vi "Report_generator.vi"() -> ()   [LabVIEW 2022 SP3]
uses:
  <vilib>/printing/EasyPrintingControls.llb/custom_contents_options.ctl
  <vilib>/printing/EasyPrintingControls.llb/list_which_controls.ctl
  <vilib>/Utility/NIReport.llb/Report Type.ctl
  <vilib>/printing/EasyPrintingControls.llb/contents.ctl
  <vilib>/Utility/NIReport.llb/Report Type (with Quick Print).ctl
  <vilib>/printing/EasyPrinting.llb/Print VI Panel or Documentation (path).vi
  <vilib>/Utility/NIReport.llb/Append Report Text (str wrap).vi
  <vilib>/printing/ReportDocExtensions.llb/Append VI Icon to Report (refnum).vi
  <vilib>/printing/ReportDocExtensions.llb/Append VI Description to Report (refnum).vi
  <vilib>/printing/ReportDocExtensions.llb/Append Front Panel Image to Report (refnum).vi
  <vilib>/printing/ReportDocExtensions.llb/Append VI List of Controls to Report (refnum).vi
  <vilib>/printing/ReportDocExtensions.llb/Append VI List of SubVIs to Report (refnum).vi
  <vilib>/printing/ReportDocExtensions.llb/Append VI Hierarchy to Report (refnum).vi
  <vilib>/Utility/NIReport.llb/NI_report.lvclass
  <vilib>/Utility/NIReport.llb/NI_ReportGenerationCore.lvlib
panel:
  out "error out 2":errorcluster
  in  "custom contents options":T1 {"list of controls options"."list which controls?" items=["all controls", "connected controls"]}
  in  "VI path":path
  out "error out":errorcluster
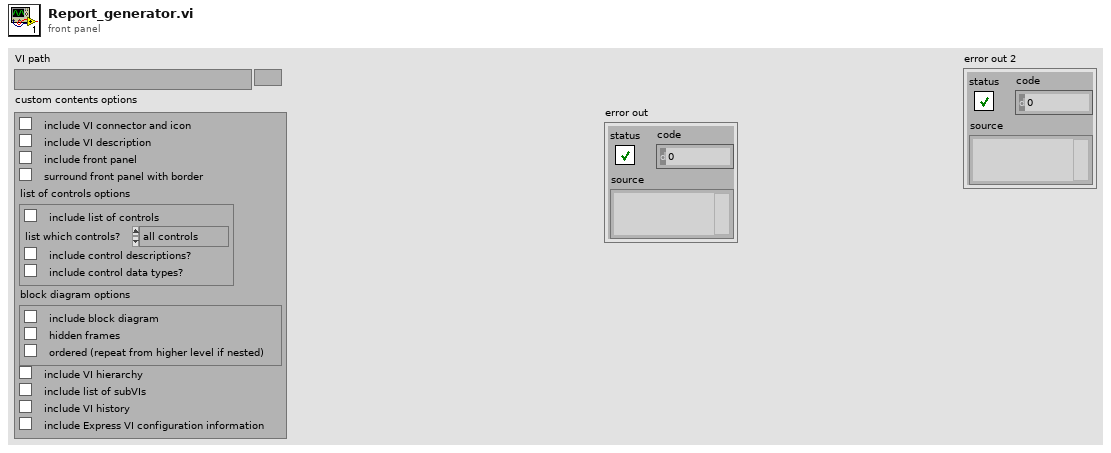
[diagram p1: front panel]
types:
  T1 = typedef "NI_ReportGenerationCore.lvlib/custom_contents_options.ctl" = cluster{"include VI connector and icon":bool, "include VI description":bool, "include front panel":bool, "surround front panel with border":bool, "list of controls options":cluster{"include list of controls":bool, "list which controls?":T2, "include control descriptions?":bool, "include control data types?":bool}, "block diagram options":cluster{"include block diagram":bool, "hidden frames":bool, "ordered (repeat from higher level if nested)":bool}, "include VI hierarchy":bool, "include list of subVIs":bool, "include VI history":bool, "include Express VI configuration information":bool}
  T2 = typedef "NI_ReportGenerationCore.lvlib/list_which_controls.ctl" = u16
  T3 = typedef "NI_ReportGenerationCore.lvlib/Report Type (with Quick Print).ctl" = enum16{"Quick Print", "HTML", "Word", "Excel"}
  T4 = typedef "NI_ReportGenerationCore.lvlib/contents.ctl" = u16
  T5 = typedef "NI_ReportGenerationCore.lvlib/Report Type.ctl" = enum16{"HTML", "Word", "Excel"}
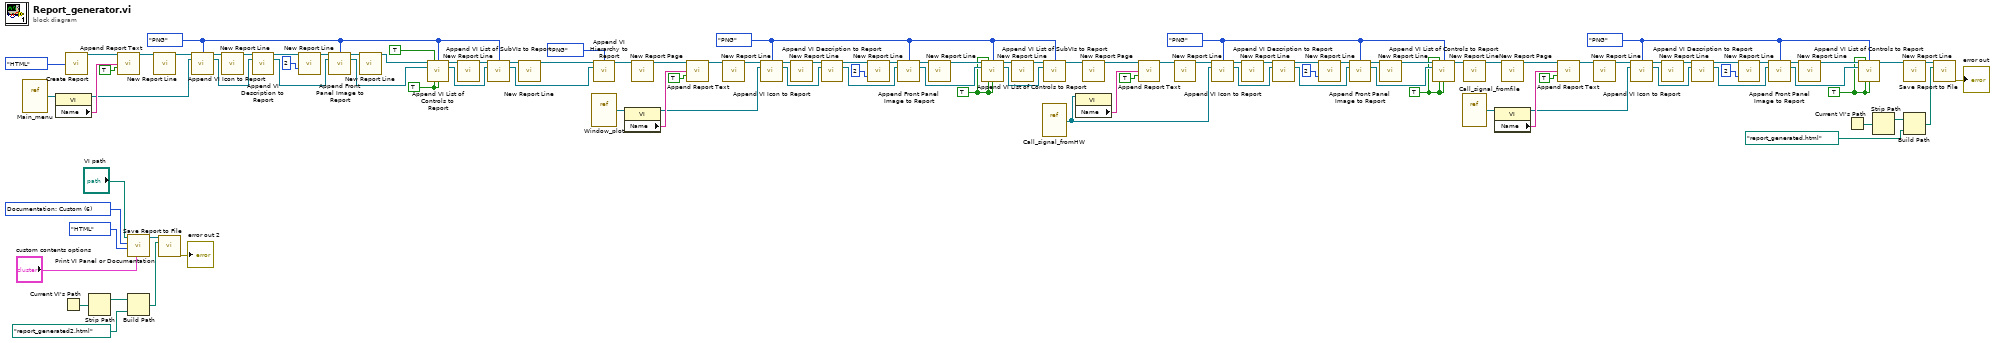
[diagram p0: block diagram]
diagram:
  w9 = T4 6 items=["Complete front panel", "Visible portion of front panel", "Icon, description, panel and diagram", "Documentation: Using the panel", "Documentation: Using as a subVI", "Documentation: Complete", "Documentation: Custom"] ("contents (complete front panel)")
  w12 = enum32{"PNG", "JPEG", "GIF"}."PNG" ("image format (jpeg)")
  w20 = TRUE ("include only controls in con pane?")
  w13 = enum32{"PNG", "JPEG", "GIF"}."PNG" ("image format (jpeg)")
  w21 = TRUE ("include only controls in con pane?")
  w14 = enum32{"PNG", "JPEG", "GIF"}."PNG" ("image format (jpeg)")
  w22 = TRUE ("include only controls in con pane?")
  w15 = enum32{"PNG", "JPEG", "GIF"}."PNG" ("image format (jpeg)")
  w23 = TRUE ("include only controls in con pane?")
  n1 = vi-ref "Main_menu.vi"() -> (w82:refnum<vi>)
  n2 = property class="VI"(reference=w82) -> (reference out=w26:refnum<vi>, "Name"=w81:string)  [unwired: 1 in, 1 out]
  n3 = Current VI's Path() -> (path=w2:path)
  n4 = call <vilib>:"Create Report.vi"("report type"=Report_Type."HTML") -> ("report out"=w107:refnum<class "NI_report.lvclass">)  [unwired: 13 in, 1 out]
  n5 = Strip Path(path=w2) -> (stripped path=w3:path)  [unwired: 1 out]
  n6 = call-poly <vilib>:"Append Report Text.vi"("report in"=w107, "text"=w81, "append on new line? (F)"=TRUE) -> ("report out"=w101:refnum<class "NI_report.lvclass">)  [unwired: 9 in, 3 out]
  n7 = call-poly <vilib>:"Print VI Panel or Documentation.vi"("custom contents options"="custom contents options", "report type (Quick Print)"=Report_Type_(with_Quick_Print)."HTML", "contents (complete front panel)"=w9, "VI path"="VI path") -> ("report out"=w1:refnum<class "NI_report.lvclass">)  [unwired: 6 in, 1 out]
  n8 = Build Path(base path=w3, name or relative path=path "report_generated2.html") -> (appended path=w5:path)
  n9 = call-dynamic "New Report Line.vi"("report in"=w101) -> ("report out"=w100:refnum<class "NI_report.lvclass">)  [unwired: 13 in, 1 out]
  n10 = call-dynamic "Save Report to File.vi"("report in"=w1, "report file path"=w5) -> ("error out"=→"error out 2":errorcluster)  [unwired: 12 in, 1 out]
  n11 = call-poly <vilib>:"Append VI Icon to Report.vi"("report in"=w100, "image format (jpeg)"=w15, "VI"=w26) -> ("report out"=w93:refnum<class "NI_report.lvclass">, "VI out"=w99:refnum<vi>)  [unwired: 8 in, 3 out]
  n12 = call-dynamic "New Report Line.vi"("report in"=w93) -> ("report out"=w94:refnum<class "NI_report.lvclass">)  [unwired: 13 in, 1 out]
  n13 = call-poly <vilib>:"Append VI Description to Report.vi"("report in"=w94, "VI"=w99) -> ("report out"=w90:refnum<class "NI_report.lvclass">, "VI out"=w98:refnum<vi>)  [unwired: 9 in, 3 out]
  n14 = call-dynamic "New Report Line.vi"("report in"=w90, "number of lines (1)"=2) -> ("report out"=w89:refnum<class "NI_report.lvclass">)  [unwired: 12 in, 1 out]
  n15 = call-poly <vilib>:"Append Front Panel Image to Report.vi"("report in"=w89, "image format (jpeg)"=w15, "VI"=w98) -> ("report out"=w92:refnum<class "NI_report.lvclass">, "VI out"=w97:refnum<vi>)  [unwired: 8 in, 3 out]
  n16 = call-dynamic "New Report Line.vi"("report in"=w92) -> ("report out"=w91:refnum<class "NI_report.lvclass">)  [unwired: 13 in, 1 out]
  n17 = call-poly <vilib>:"Append VI List of Controls to Report.vi"("report in"=w91, "include only controls in con pane?"=TRUE, "image format (jpeg)"=w15, "VI"=w97, "include control descriptions?"=w23, "include control data types?"=w23) -> ("report out"=w87:refnum<class "NI_report.lvclass">, "VI out"=w96:refnum<vi>)  [unwired: 5 in, 3 out]
  n18 = call-dynamic "New Report Line.vi"("report in"=w87) -> ("report out"=w86:refnum<class "NI_report.lvclass">)  [unwired: 13 in, 1 out]
  n19 = call-poly <vilib>:"Append VI List of SubVIs to Report.vi"("report in"=w86, "image format (jpeg)"=w15, "VI"=w96) -> ("report out"=w85:refnum<class "NI_report.lvclass">, "VI out"=w95:refnum<vi>)  [unwired: 8 in, 3 out]
  n20 = call-dynamic "New Report Line.vi"("report in"=w85) -> ("report out"=w84:refnum<class "NI_report.lvclass">)  [unwired: 13 in, 1 out]
  n21 = vi-ref "Window_plot.vi"() -> (w62:refnum<vi>)
  n22 = call-poly <vilib>:"Append VI Hierarchy to Report.vi"("report in"=w84, "image format (jpeg)"=enum32{"PNG", "JPEG", "GIF"}."PNG", "VI"=w95) -> ("report out"=w83:refnum<class "NI_report.lvclass">)  [unwired: 8 in, 4 out]
  n23 = property class="VI"(reference=w62) -> (reference out=w27:refnum<vi>, "Name"=w80:string)  [unwired: 1 in, 1 out]
  n24 = call-dynamic "New Report Page.vi"("report in"=w83) -> ("report out"=w63:refnum<class "NI_report.lvclass">)  [unwired: 13 in, 1 out]
  n25 = call-poly <vilib>:"Append Report Text.vi"("report in"=w63, "text"=w80, "append on new line? (F)"=TRUE) -> ("report out"=w65:refnum<class "NI_report.lvclass">)  [unwired: 9 in, 3 out]
  n26 = call-dynamic "New Report Line.vi"("report in"=w65) -> ("report out"=w66:refnum<class "NI_report.lvclass">)  [unwired: 13 in, 1 out]
  n27 = call-poly <vilib>:"Append VI Icon to Report.vi"("report in"=w66, "image format (jpeg)"=w14, "VI"=w27) -> ("report out"=w72:refnum<class "NI_report.lvclass">, "VI out"=w67:refnum<vi>)  [unwired: 8 in, 3 out]
  n28 = call-dynamic "New Report Line.vi"("report in"=w72) -> ("report out"=w71:refnum<class "NI_report.lvclass">)  [unwired: 13 in, 1 out]
  n29 = call-poly <vilib>:"Append VI Description to Report.vi"("report in"=w71, "VI"=w67) -> ("report out"=w75:refnum<class "NI_report.lvclass">, "VI out"=w68:refnum<vi>)  [unwired: 9 in, 3 out]
  n30 = call-dynamic "New Report Line.vi"("report in"=w75, "number of lines (1)"=2) -> ("report out"=w76:refnum<class "NI_report.lvclass">)  [unwired: 12 in, 1 out]
  n31 = call-poly <vilib>:"Append Front Panel Image to Report.vi"("report in"=w76, "image format (jpeg)"=w14, "VI"=w68) -> ("report out"=w73:refnum<class "NI_report.lvclass">, "VI out"=w69:refnum<vi>)  [unwired: 8 in, 3 out]
  n32 = call-dynamic "New Report Line.vi"("report in"=w73) -> ("report out"=w74:refnum<class "NI_report.lvclass">)  [unwired: 13 in, 1 out]
  n33 = call-poly <vilib>:"Append VI List of Controls to Report.vi"("report in"=w74, "include only controls in con pane?"=w22, "image format (jpeg)"=w14, "VI"=w69, "include control descriptions?"=w22, "include control data types?"=w22) -> ("report out"=w78:refnum<class "NI_report.lvclass">, "VI out"=w70:refnum<vi>)  [unwired: 5 in, 3 out]
  n34 = call-dynamic "New Report Line.vi"("report in"=w78) -> ("report out"=w79:refnum<class "NI_report.lvclass">)  [unwired: 13 in, 1 out]
  n35 = vi-ref "Call_signal_fromHW.vi"() -> (w46:refnum<vi>)
  n36 = call-poly <vilib>:"Append VI List of SubVIs to Report.vi"("report in"=w79, "image format (jpeg)"=w14, "VI"=w70) -> ("report out"=w16:refnum<class "NI_report.lvclass">)  [unwired: 8 in, 4 out]
  n37 = property class="VI"(reference=w46) -> ("Name"=w47:string)  [unwired: 1 in, 2 out]
  n38 = call-dynamic "New Report Page.vi"("report in"=w16) -> ("report out"=w30:refnum<class "NI_report.lvclass">)  [unwired: 13 in, 1 out]
  n39 = call-poly <vilib>:"Append Report Text.vi"("report in"=w30, "text"=w47, "append on new line? (F)"=TRUE) -> ("report out"=w60:refnum<class "NI_report.lvclass">)  [unwired: 9 in, 3 out]
  n40 = call-dynamic "New Report Line.vi"("report in"=w60) -> ("report out"=w59:refnum<class "NI_report.lvclass">)  [unwired: 13 in, 1 out]
  n41 = call-poly <vilib>:"Append VI Icon to Report.vi"("report in"=w59, "image format (jpeg)"=w13, "VI"=w46) -> ("report out"=w54:refnum<class "NI_report.lvclass">, "VI out"=w58:refnum<vi>)  [unwired: 8 in, 3 out]
  n42 = call-dynamic "New Report Line.vi"("report in"=w54) -> ("report out"=w55:refnum<class "NI_report.lvclass">)  [unwired: 13 in, 1 out]
  n43 = call-poly <vilib>:"Append VI Description to Report.vi"("report in"=w55, "VI"=w58) -> ("report out"=w51:refnum<class "NI_report.lvclass">, "VI out"=w57:refnum<vi>)  [unwired: 9 in, 3 out]
  n44 = call-dynamic "New Report Line.vi"("report in"=w51, "number of lines (1)"=2) -> ("report out"=w50:refnum<class "NI_report.lvclass">)  [unwired: 12 in, 1 out]
  n45 = call-poly <vilib>:"Append Front Panel Image to Report.vi"("report in"=w50, "image format (jpeg)"=w13, "VI"=w57) -> ("report out"=w53:refnum<class "NI_report.lvclass">, "VI out"=w56:refnum<vi>)  [unwired: 8 in, 3 out]
  n46 = call-dynamic "New Report Line.vi"("report in"=w53) -> ("report out"=w52:refnum<class "NI_report.lvclass">)  [unwired: 13 in, 1 out]
  n47 = call-poly <vilib>:"Append VI List of Controls to Report.vi"("report in"=w52, "include only controls in con pane?"=w21, "image format (jpeg)"=w13, "VI"=w56, "include control descriptions?"=w21, "include control data types?"=w21) -> ("report out"=w48:refnum<class "NI_report.lvclass">)  [unwired: 5 in, 4 out]
  n48 = vi-ref "Call_signal_fromfile.vi"() -> (w29:refnum<vi>)
  n49 = call-dynamic "New Report Line.vi"("report in"=w48) -> ("report out"=w19:refnum<class "NI_report.lvclass">)  [unwired: 13 in, 1 out]
  n50 = property class="VI"(reference=w29) -> (reference out=w25:refnum<vi>, "Name"=w45:string)  [unwired: 1 in, 1 out]
  n51 = call-dynamic "New Report Page.vi"("report in"=w19) -> ("report out"=w28:refnum<class "NI_report.lvclass">)  [unwired: 13 in, 1 out]
  n52 = call-poly <vilib>:"Append Report Text.vi"("report in"=w28, "text"=w45, "append on new line? (F)"=TRUE) -> ("report out"=w32:refnum<class "NI_report.lvclass">)  [unwired: 9 in, 3 out]
  n53 = call-dynamic "New Report Line.vi"("report in"=w32) -> ("report out"=w33:refnum<class "NI_report.lvclass">)  [unwired: 13 in, 1 out]
  n54 = call-poly <vilib>:"Append VI Icon to Report.vi"("report in"=w33, "image format (jpeg)"=w12, "VI"=w25) -> ("report out"=w38:refnum<class "NI_report.lvclass">, "VI out"=w34:refnum<vi>)  [unwired: 8 in, 3 out]
  n55 = call-dynamic "New Report Line.vi"("report in"=w38) -> ("report out"=w37:refnum<class "NI_report.lvclass">)  [unwired: 13 in, 1 out]
  n56 = call-poly <vilib>:"Append VI Description to Report.vi"("report in"=w37, "VI"=w34) -> ("report out"=w41:refnum<class "NI_report.lvclass">, "VI out"=w35:refnum<vi>)  [unwired: 9 in, 3 out]
  n57 = call-dynamic "New Report Line.vi"("report in"=w41, "number of lines (1)"=2) -> ("report out"=w42:refnum<class "NI_report.lvclass">)  [unwired: 12 in, 1 out]
  n58 = call-poly <vilib>:"Append Front Panel Image to Report.vi"("report in"=w42, "image format (jpeg)"=w12, "VI"=w35) -> ("report out"=w39:refnum<class "NI_report.lvclass">, "VI out"=w36:refnum<vi>)  [unwired: 8 in, 3 out]
  n59 = call-dynamic "New Report Line.vi"("report in"=w39) -> ("report out"=w40:refnum<class "NI_report.lvclass">)  [unwired: 13 in, 1 out]
  n60 = Current VI's Path() -> (path=w106:path)
  n61 = call-poly <vilib>:"Append VI List of Controls to Report.vi"("report in"=w40, "include only controls in con pane?"=w20, "image format (jpeg)"=w12, "VI"=w36, "include control descriptions?"=w20, "include control data types?"=w20) -> ("report out"=w44:refnum<class "NI_report.lvclass">)  [unwired: 5 in, 4 out]
  n62 = Strip Path(path=w106) -> (stripped path=w105:path)  [unwired: 1 out]
  n63 = call-dynamic "New Report Line.vi"("report in"=w44) -> ("report out"=w24:refnum<class "NI_report.lvclass">)  [unwired: 13 in, 1 out]
  n64 = Build Path(base path=w105, name or relative path=path "report_generated.html") -> (appended path=w103:path)
  n65 = call-dynamic "Save Report to File.vi"("report in"=w24, "report file path"=w103) -> ("error out"=→"error out":errorcluster)  [unwired: 12 in, 1 out]
